vi "Gryro Math Calc.vi"(8 "Reset Integrator":bool, 9 "Temperature (Pure doule precision HW) in":dbl, 10 "Gyroscopic Cluster Values In":dbl[](array[numeric]), 11 "Accel Array":dbl[](array[numeric])) -> (0 "Temperature (Scaled) out":dbl, 1 "Linear Acceleration [LSB/sec^2]":dbl[](array[numeric]), 2 "Angular Displacement (Gyro)":dbl[](array[numeric]), 3 "Angular Gyro Rate [LSB/sec]":dbl[](array[numeric]))   [LabVIEW 2014]
uses:
  Globals_Real.vi
  <vilib>/ptbypt/NI_PtbyPt.lvlib
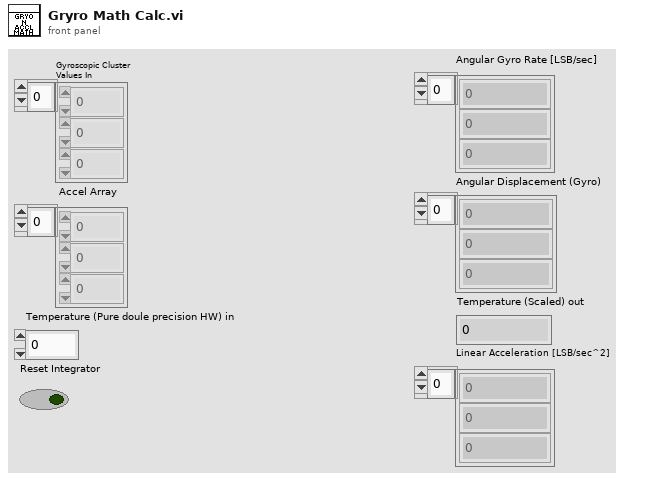
[diagram p1: front panel]
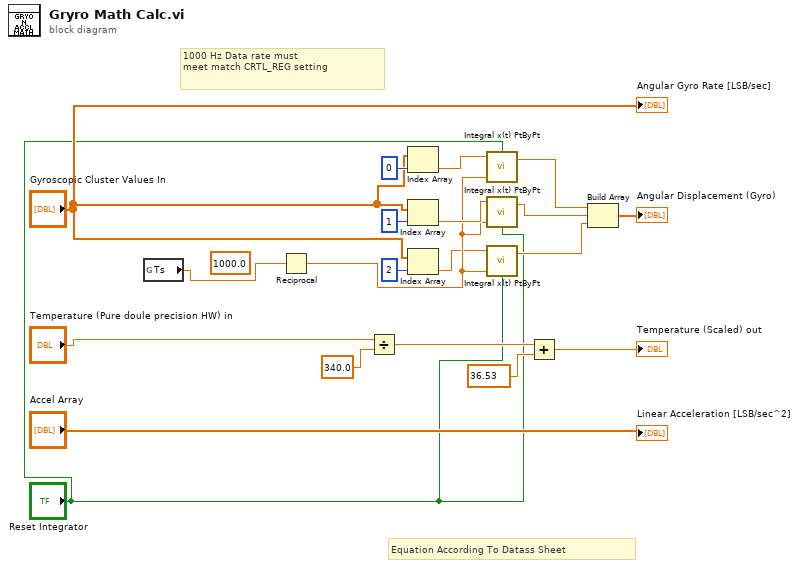
[diagram p0: block diagram]
diagram:
  (unwired) 1000.0 ("dt")
  # "Equation According To Datass Sheet"
  # "1000 Hz Data rate must\nmeet match CRTL_REG setting"
  n1 = global read "Globals_Real.vi" "Ts"() -> (w1:dbl)
  n2 = Reciprocal(x=w1) -> (1/x=w4:dbl)
  n3 = Divide(x="Temperature (Pure doule precision HW) in", y=340.0) -> (x/y=w18:dbl)
  n4 = Index Array(array="Gyroscopic Cluster Values In", index=0) -> (element=w14:dbl)
  n5 = Index Array(array="Gyroscopic Cluster Values In", index=1) -> (element=w8:dbl)
  n6 = Index Array(array="Gyroscopic Cluster Values In", index=2) -> (element=w3:dbl)
  n7 = call <vilib>:"Integral x(t) PtByPt.vi"("initialize"="Reset Integrator", "dt"=w4, "x"=w14) -> ("integral x(t)"=w13:dbl)  [unwired: 1 in, 1 out]
  n8 = call <vilib>:"Integral x(t) PtByPt.vi"("initialize"="Reset Integrator", "dt"=w4, "x"=w8) -> ("integral x(t)"=w10:dbl)  [unwired: 1 in, 1 out]
  n9 = call <vilib>:"Integral x(t) PtByPt.vi"("initialize"="Reset Integrator", "dt"=w4, "x"=w3) -> ("integral x(t)"=w9:dbl)  [unwired: 1 in, 1 out]
  n10 = Add(x=w18, y=36.53) -> (x+y=→"Temperature (Scaled) out":dbl)
  n11 = Build Array(w13, w10, w9) -> (→"Angular Displacement (Gyro)":dbl[])
  "Angular Gyro Rate [LSB/sec]" <- "Gyroscopic Cluster Values In"
  "Linear Acceleration [LSB/sec^2]" <- "Accel Array"
